vi "Enqueue Sample.vi"(0 "Sift Client in":refnum<class "Sift Client.lvclass">, 1 "Values":variant[](array[variant]), 3 "Timestamp":T2, 4 "Flow Name":string, 5 "error in (no error)":errorcluster, 7 "Data Type":T12) -> (14 "Sift Client out":refnum<class "Sift Client.lvclass">, 19 "error out":errorcluster)   [LabVIEW 2024, in "Sift Client.lvlib" / "Sift Client.lvclass"]
doc: "Add a sample of data for the specified flow to the data queue."
uses:
  Sift Client.lvclass
  Generate Sift Protos/SiftProxy_client/RPC Messages/sift_proxy_v1_ChannelDataType.ctl
  Typedefs/Double Sample.ctl
  Generate Sift Protos/SiftProxy_client/RPC Messages/google_protobuf_Timestamp.ctl
  Typedefs/String Sample.ctl
  Typedefs/Enum Sample.ctl
  Typedefs/Bitfield Sample.ctl
  Typedefs/Bool Sample.ctl
  Typedefs/Float Sample.ctl
  Typedefs/Int32 Sample.ctl
  Typedefs/Int64 Sample.ctl
  Typedefs/Uint32 Sample.ctl
  Typedefs/Uint64 Sample.ctl
  Sift Client.lvclass/Sift Client.ctl
  Generate Sift Protos/SiftProxy_client/SiftProxy_client.lvlib
  Sift Client.lvlib
panel:
  in  "Uint64 Sample":T1
  in  "Uint32 Sample":T3
  in  "Int64 Sample":T4
  in  "Int32 Sample":T5
  in  "Float Sample":T6
  in  "Bool Sample":T7
  in  "Bitfield Sample":T8
  in  "Enum Sample":T9
  in  "String Sample":T10
  in  "Double Sample":T11
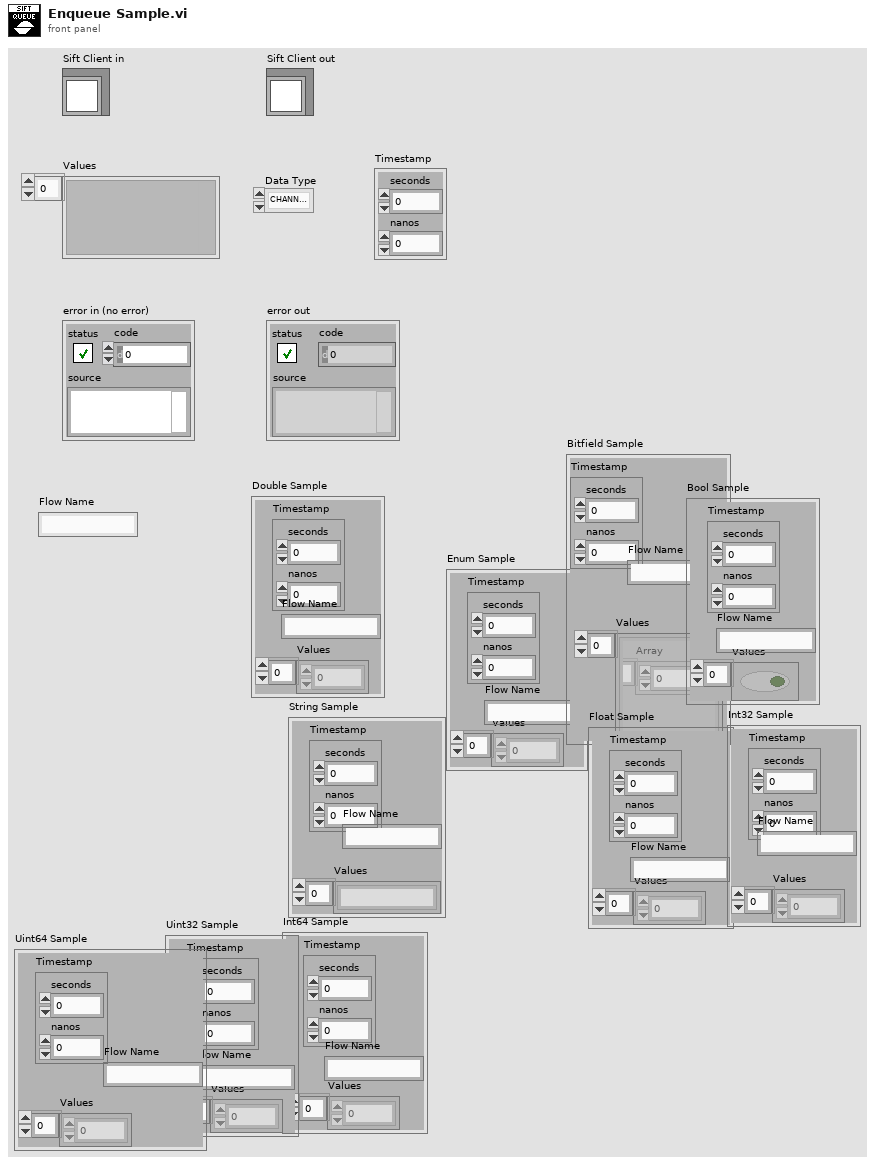
[diagram p1: front panel]
types:
  T1 = typedef "Sift Client.lvlib/Uint64 Sample.ctl" = cluster{"Values":u64[], "Timestamp":T2, "Flow Name":string}
  T2 = typedef "SiftProxy_client.lvlib/google_protobuf_Timestamp.ctl" = cluster{"seconds":i64, "nanos":i32}
  T3 = typedef "Sift Client.lvlib/Uint32 Sample.ctl" = cluster{"Values":u32[], "Timestamp":T2, "Flow Name":string}
  T4 = typedef "Sift Client.lvlib/Int64 Sample.ctl" = cluster{"Values":i64[], "Timestamp":T2, "Flow Name":string}
  T5 = typedef "Sift Client.lvlib/Int32 Sample.ctl" = cluster{"Values":i32[], "Timestamp":T2, "Flow Name":string}
  T6 = typedef "Sift Client.lvlib/Float Sample.ctl" = cluster{"Values":sgl[], "Timestamp":T2, "Flow Name":string}
  T7 = typedef "Sift Client.lvlib/Bool Sample.ctl" = cluster{"Values":bool[], "Timestamp":T2, "Flow Name":string}
  T8 = typedef "Sift Client.lvlib/Bitfield Sample.ctl" = cluster{"Timestamp":T2, "Values":cluster{"Array":u8[]}[], "Flow Name":string}
  T9 = typedef "Sift Client.lvlib/Enum Sample.ctl" = cluster{"Values":u32[], "Timestamp":T2, "Flow Name":string}
  T10 = typedef "Sift Client.lvlib/String Sample.ctl" = cluster{"Values":string[], "Timestamp":T2, "Flow Name":string}
  T11 = typedef "Sift Client.lvlib/Double Sample.ctl" = cluster{"Values":dbl[], "Timestamp":T2, "Flow Name":string}
  T12 = typedef "SiftProxy_client.lvlib/sift_proxy_v1_ChannelDataType.ctl" = enum32{"CHANNEL_DATA_TYPE_UNSPECIFIED", "CHANNEL_DATA_TYPE_DOUBLE", "CHANNEL_DATA_TYPE_STRING", "CHANNEL_DATA_TYPE_ENUM", "CHANNEL_DATA_TYPE_BIT_FIELD", "CHANNEL_DATA_TYPE_BOOL", "CHANNEL_DATA_TYPE_FLOAT", "CHANNEL_DATA_TYPE_INT_32", "CHANNEL_DATA_TYPE_UINT_32", "CHANNEL_DATA_TYPE_INT_64", "CHANNEL_DATA_TYPE_UINT_64"}
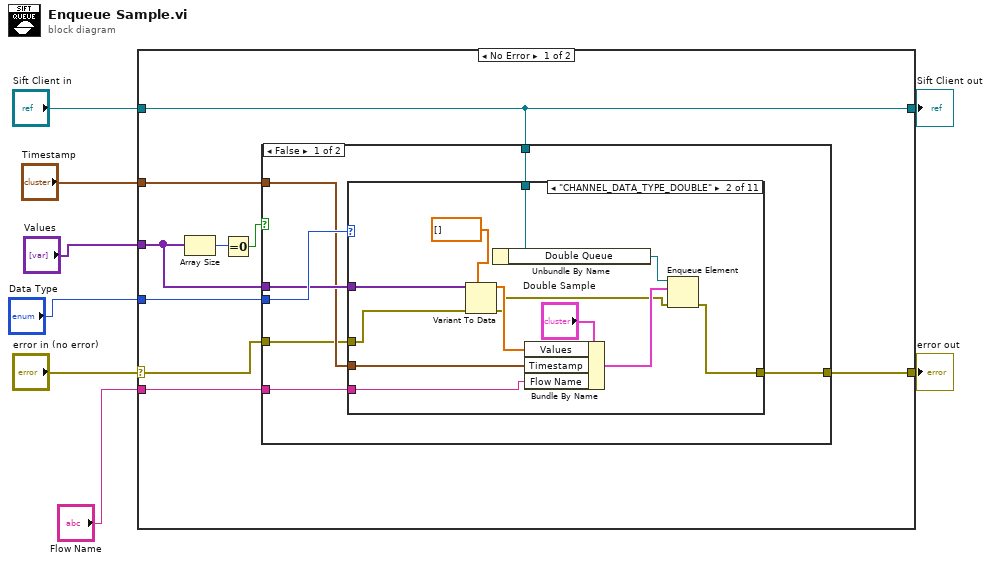
[diagram p0: block diagram]
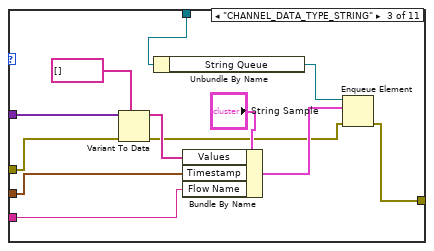
[diagram p3: hidden frame]
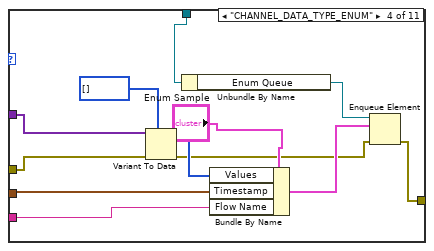
[diagram p4: hidden frame]
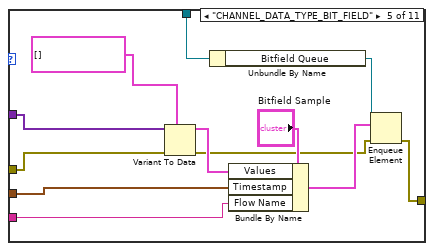
[diagram p5: hidden frame]
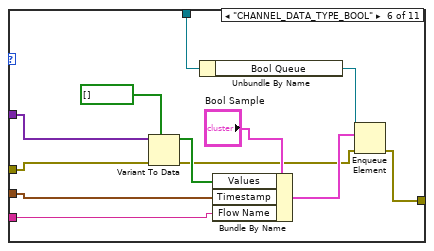
[diagram p6: hidden frame]
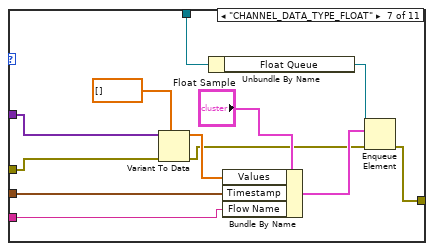
[diagram p7: hidden frame]
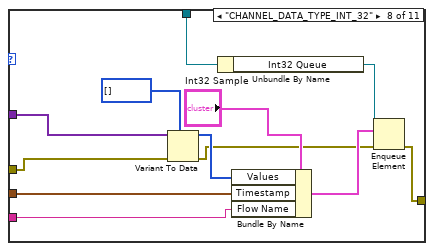
[diagram p8: hidden frame]
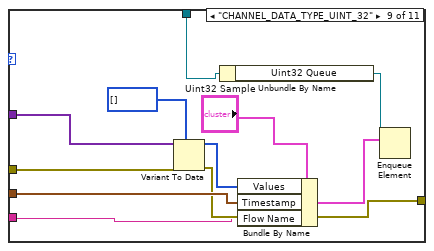
[diagram p9: hidden frame]
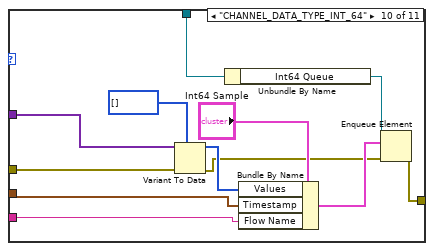
[diagram p10: hidden frame]
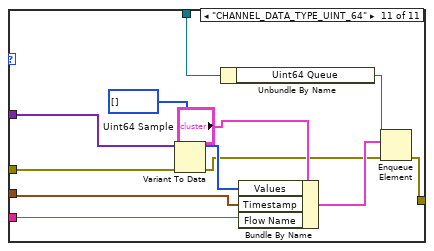
[diagram p11: hidden frame]
diagram:
  n1 = case shown="No Error" "error in (no error)" {
    selector: "error in (no error)" -> [w11 w147]
    tunnel: [w10 w147] -> w7
    tunnel: [w13 w146] -> w5
    tunnel: "Sift Client in" -> [w13 w146]
    tunnel: "Values" -> [w14 _]
    tunnel: "Data Type" -> [w15 _]
    tunnel: "Timestamp" -> [w12 _]
    tunnel: "Flow Name" -> [w9 _]
    frame No Error {
      n2 = Array Size(array=w14) -> (size(s)=w17:i32)
      n3 = Equal To 0?(x=w17) -> (x = 0?=w16:bool)
      n4 = case shown="False" w16 {
        tunnel: w15 -> [w24 _]
        tunnel: w14 -> [w23 _]
        tunnel: w13 -> [w21 _]
        tunnel: w12 -> [w22 _]
        tunnel: w11 -> [w20 w145]
        tunnel: [w19 w145] -> w10
        tunnel: w9 -> [w18 _]
        frame False {
          n5 = case shown="\"CHANNEL_DATA_TYPE_DOUBLE\"" w24 {
            tunnel: w23 -> [_ w36 w43 w54 w67 w78 w90 w104 w115 w127 w139]
            tunnel: w21 -> [_ w35 w42 w57 w68 w79 w91 w103 w116 w126 w138]
            tunnel: w22 -> [_ w34 w45 w56 w70 w80 w93 w105 w114 w128 w140]
            tunnel: w20 -> [w25 w29 w41 w53 w66 w77 w89 w101 w112 w124 w136]
            tunnel: [w25 w27 w39 w51 w64 w75 w87 w99 w111 w122 w134] -> w19
            tunnel: w18 -> [_ w26 w38 w50 w62 w74 w86 w98 w110 w121 w133]
            frame "CHANNEL_DATA_TYPE_UNSPECIFIED", Default {
            }
            frame "CHANNEL_DATA_TYPE_DOUBLE" {
              n6 = Variant To Data(error in=w29, type=dbl[] [], Variant=w36) -> (data=w33:dbl[], error out=w28:errorcluster)
              n7 = Unbundle By Name(w35) -> ("Double Queue"=w30:refnum<queue>)
              n8 = Bundle By Name(cluster="Double Sample", "Values"=w33, "Timestamp"=w34, "Flow Name"=w26) -> (w31:T11)
              n9 = Enqueue Element(queue=w30, element=w31, error in (no error)=w28) -> (error out=w27:errorcluster)  [unwired: 1 in, 2 out]
            }
            frame "CHANNEL_DATA_TYPE_STRING" {
              n10 = Variant To Data(error in=w41, type=string[] [], Variant=w43) -> (data=w48:string[], error out=w40:errorcluster)
              n11 = Unbundle By Name(w42) -> ("String Queue"=w46:refnum<queue>)
              n12 = Bundle By Name(cluster="String Sample", "Values"=w48, "Timestamp"=w45, "Flow Name"=w38) -> (w47:T10)
              n13 = Enqueue Element(queue=w46, element=w47, error in (no error)=w40) -> (error out=w39:errorcluster)  [unwired: 1 in, 2 out]
            }
            frame "CHANNEL_DATA_TYPE_ENUM" {
              n14 = Variant To Data(error in=w53, type=u32[] [], Variant=w54) -> (data=w60:u32[], error out=w52:errorcluster)
              n15 = Unbundle By Name(w57) -> ("Enum Queue"=w58:refnum<queue>)
              n16 = Bundle By Name(cluster="Enum Sample", "Values"=w60, "Timestamp"=w56, "Flow Name"=w50) -> (w59:T9)
              n17 = Enqueue Element(queue=w58, element=w59, error in (no error)=w52) -> (error out=w51:errorcluster)  [unwired: 1 in, 2 out]
            }
            frame "CHANNEL_DATA_TYPE_BIT_FIELD" {
              n18 = Variant To Data(error in=w66, type=cluster{u8[]}[] [], Variant=w67) -> (data=w73:cluster{u8[]}[], error out=w65:errorcluster)
              n19 = Unbundle By Name(w68) -> ("Bitfield Queue"=w71:refnum<queue>)
              n20 = Bundle By Name(cluster="Bitfield Sample", "Values"=w73, "Timestamp"=w70, "Flow Name"=w62) -> (w72:T8)
              n21 = Enqueue Element(queue=w71, element=w72, error in (no error)=w65) -> (error out=w64:errorcluster)  [unwired: 1 in, 2 out]
            }
            frame "CHANNEL_DATA_TYPE_BOOL" {
              n22 = Variant To Data(error in=w77, type=bool[] [], Variant=w78) -> (data=w84:bool[], error out=w76:errorcluster)
              n23 = Unbundle By Name(w79) -> ("Bool Queue"=w82:refnum<queue>)
              n24 = Bundle By Name(cluster="Bool Sample", "Values"=w84, "Timestamp"=w80, "Flow Name"=w74) -> (w83:T7)
              n25 = Enqueue Element(queue=w82, element=w83, error in (no error)=w76) -> (error out=w75:errorcluster)  [unwired: 1 in, 2 out]
            }
            frame "CHANNEL_DATA_TYPE_FLOAT" {
              n26 = Variant To Data(error in=w89, type=sgl[] [], Variant=w90) -> (data=w96:sgl[], error out=w88:errorcluster)
              n27 = Unbundle By Name(w91) -> ("Float Queue"=w94:refnum<queue>)
              n28 = Bundle By Name(cluster="Float Sample", "Values"=w96, "Timestamp"=w93, "Flow Name"=w86) -> (w95:T6)
              n29 = Enqueue Element(queue=w94, element=w95, error in (no error)=w88) -> (error out=w87:errorcluster)  [unwired: 1 in, 2 out]
            }
            frame "CHANNEL_DATA_TYPE_INT_32" {
              n30 = Variant To Data(error in=w101, type=i32[] [], Variant=w104) -> (data=w108:i32[], error out=w100:errorcluster)
              n31 = Unbundle By Name(w103) -> ("Int32 Queue"=w106:refnum<queue>)
              n32 = Bundle By Name(cluster="Int32 Sample", "Values"=w108, "Timestamp"=w105, "Flow Name"=w98) -> (w107:T5)
              n33 = Enqueue Element(queue=w106, element=w107, error in (no error)=w100) -> (error out=w99:errorcluster)  [unwired: 1 in, 2 out]
            }
            frame "CHANNEL_DATA_TYPE_UINT_32" {
              n34 = Variant To Data(error in=w112, type=u32[] [], Variant=w115) -> (data=w119:u32[], error out=w111:errorcluster)
              n35 = Unbundle By Name(w116) -> ("Uint32 Queue"=w117:refnum<queue>)
              n36 = Bundle By Name(cluster="Uint32 Sample", "Values"=w119, "Timestamp"=w114, "Flow Name"=w110) -> (w118:T3)
              n37 = Enqueue Element(queue=w117, element=w118) -> ()  [unwired: 2 in, 3 out]
            }
            frame "CHANNEL_DATA_TYPE_INT_64" {
              n38 = Variant To Data(error in=w124, type=i64[] [], Variant=w127) -> (data=w131:i64[], error out=w123:errorcluster)
              n39 = Unbundle By Name(w126) -> ("Int64 Queue"=w129:refnum<queue>)
              n40 = Bundle By Name(cluster="Int64 Sample", "Values"=w131, "Timestamp"=w128, "Flow Name"=w121) -> (w130:T4)
              n41 = Enqueue Element(queue=w129, element=w130, error in (no error)=w123) -> (error out=w122:errorcluster)  [unwired: 1 in, 2 out]
            }
            frame "CHANNEL_DATA_TYPE_UINT_64" {
              n42 = Variant To Data(error in=w136, type=i64[] [], Variant=w139) -> (data=w143:i64[], error out=w135:errorcluster)
              n43 = Unbundle By Name(w138) -> ("Uint64 Queue"=w141:refnum<queue>)
              n44 = Bundle By Name(cluster="Uint64 Sample", "Values"=w143, "Timestamp"=w140, "Flow Name"=w133) -> (w142:T1)
              n45 = Enqueue Element(queue=w141, element=w142, error in (no error)=w135) -> (error out=w134:errorcluster)  [unwired: 1 in, 2 out]
            }
          }
        }
        frame True {
        }
      }
    }
    frame Error {
    }
  }
  "error out" <- w7
  "Sift Client out" <- w5
